vi "IsInBounds.vi"(9 "Vertical":i32, 10 "Horizontal":i32, 11 "ListBox in":refnum<vi>) -> (3 "Boolean":bool)   [LabVIEW 2017, in "DisplayWindow.lvlib" / "DisplayWindow.lvclass"]
uses:
  DisplayWindow.lvclass
panel:
  out "error out":errorcluster
  in  "error in (no error)":errorcluster
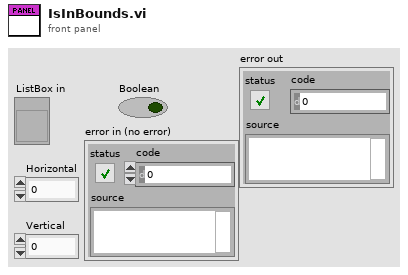
[diagram p1: front panel]
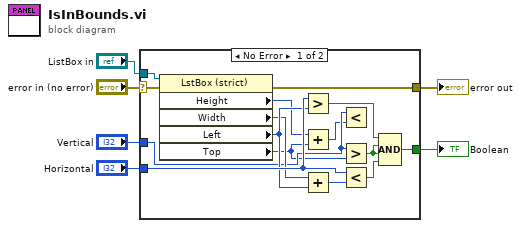
[diagram p0: block diagram]
diagram:
  n1 = case shown="No Error" "error in (no error)" {
    selector: "error in (no error)" -> [w7 w22]
    tunnel: "Horizontal" -> [w19 _]
    tunnel: "Vertical" -> [w15 _]
    tunnel: [w10 _] -> w4
    tunnel: "ListBox in" -> [w9 _]
    tunnel: [w8 w22] -> w2
    frame No Error {
      n2 = property on="Property Node" class="LstBox (strict)"(reference=w9, error in=w7) -> (error out=w8:errorcluster, "Height"=w12:u32, "Width"=w16:u32, "Left"=w17:i32, "Top"=w13:i32)  [unwired: 1 out]
      n3 = Greater?(x=w19, y=w17) -> (0:w11:bool)
      n4 = Add(x=w12, y=w13) -> (x+y=w14:u32)
      n5 = Add(x=w16, y=w17) -> (x+y=w18:u32)
      n6 = Less?(x=w15, y=w14) -> ()  [unwired: 1 out]
      n7 = Greater?(x=w15, y=w13) -> (0:w21:bool)
      n8 = Less?(x=w19, y=w18) -> (x < y?=w20:bool)
      n9 = Compound Arithmetic op=AND(w11, w21, w21, w20) -> (w10:bool)
    }
    frame Error {
    }
  }
  "Boolean" <- w4
  "error out" <- w2
